vi "3D Hydrogen.vi"(9 "Z-Position":dbl format="%#_13g") -> (1 "reference out":refnum<vi>)   [LabVIEW 2023]
uses:
  <vilib>/picture/3D Picture Control/Object/Create Object (name).vi
  <vilib>/picture/3D Picture Control/Object/Add Object (no reference).vi
  <vilib>/picture/3D Picture Control/NI_3D Picture Control.lvlib
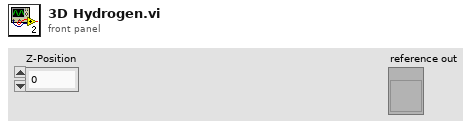
[diagram p1: front panel]
types:
  T1 = cluster{"Red":sgl, "Green":sgl, "Blue":sgl, "Alpha":sgl}
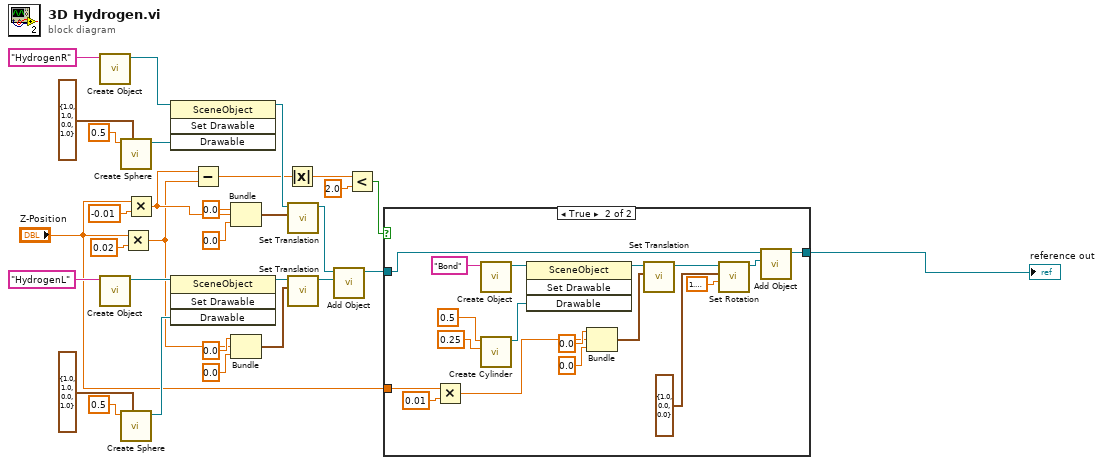
[diagram p0: block diagram]
diagram:
  n1 = call-poly <vilib>:"Create Object.vi"("Name"="HydrogenR") -> ("Scene:New Object"=w29:refnum<vi>)  [unwired: 9 in, 1 out]
  n2 = call-poly <vilib>:"Create Object.vi"("Name"="HydrogenL") -> ("Scene:New Object"=w24:refnum<vi>)  [unwired: 9 in, 1 out]
  n3 = call <vilib>:"Create Sphere.vi"("Color"=T1 {"Red"=1.0, "Green"=1.0, "Blue"=0.0, "Alpha"=1.0}, "Radius"=sgl 0.5) -> ("New Sphere Refnum"=w27:refnum<vi>)  [unwired: 8 in, 1 out]
  n4 = call <vilib>:"Create Sphere.vi"("Color"=T1 {"Red"=1.0, "Green"=1.0, "Blue"=0.0, "Alpha"=1.0}, "Radius"=sgl 0.5) -> ("New Sphere Refnum"=w22:refnum<vi>)  [unwired: 8 in, 1 out]
  n5 = Multiply(x="Z-Position", y=0.02) -> (x*y=w1:dbl)
  n6 = Multiply(x="Z-Position", y=-0.01) -> (x*y=w3:dbl)
  n7 = invoke class="SceneObject" method="Set Drawable"(reference=w29, "Drawable"=w27) -> (reference out=w13:refnum<vi>)  [unwired: 2 in, 3 out]
  n8 = invoke class="SceneObject" method="Set Drawable"(reference=w24, "Drawable"=w22) -> (reference out=w21:refnum<vi>)  [unwired: 2 in, 3 out]
  n9 = Subtract(x=w3, y=w1) -> (x-y=w6:dbl)
  n10 = Bundle(0.0, w3, 0.0) -> (w16:cluster{dbl, dbl, dbl})  [unwired: 1 in]
  n11 = Bundle(0.0, w1, 0.0) -> (w19:cluster{dbl, dbl, dbl})  [unwired: 1 in]
  n12 = Absolute Value(x=w6) -> (abs(x)=w8:dbl)
  n13 = call <vilib>:"Set Translation.vi"("Translation"=w16, "Scene Object"=w13) -> ("Translated Object"=w12:refnum<vi>)  [unwired: 8 in, 1 out]
  n14 = call <vilib>:"Set Translation.vi"("Translation"=w19, "Scene Object"=w21) -> ("Translated Object"=w20:refnum<vi>)  [unwired: 8 in, 1 out]
  n15 = call-poly <vilib>:"Add Object.vi"("New Object In"=w20, "Scene Object In"=w12) -> ("Scene Object Out"=w11:refnum<vi>)  [unwired: 8 in, 1 out]
  n16 = Less?(x=w8, y=2.0) -> (x < y?=w9:bool)
  n17 = case shown="True" w9 {
    tunnel: [w32 w44] -> w5
    tunnel: w11 -> [w32 w41]
    tunnel: "Z-Position" -> [_ w36]
    frame False {
    }
    frame True {
      n18 = Multiply(x=w36, y=0.01) -> (x*y=w33:dbl)
      n19 = call-poly <vilib>:"Create Object.vi"("Name"="Bond") -> ("Scene:New Object"=w49:refnum<vi>)  [unwired: 9 in, 1 out]
      n20 = call <vilib>:"Create Cylinder.vi"("Radius"=sgl 0.25, "Height"=sgl 0.5) -> ("New Cylinder Refnum"=w50:refnum<vi>)  [unwired: 8 in, 1 out]
      n21 = invoke class="SceneObject" method="Set Drawable"(reference=w49, "Drawable"=w50) -> (reference out=w45:refnum<vi>)  [unwired: 2 in, 3 out]
      n22 = Bundle(0.0, w33, 0.0) -> (w37:cluster{dbl, dbl, dbl})  [unwired: 1 in]
      n23 = call <vilib>:"Set Translation.vi"("Translation"=w37, "Scene Object"=w45) -> ("Translated Object"=w40:refnum<vi>)  [unwired: 8 in, 1 out]
      n24 = call <vilib>:"Set Rotation.vi"("Angle"=1.5707963267948966, "Axis"=cluster{"X":sgl, "Y":sgl, "Z":sgl} {"X"=1.0, "Y"=0.0, "Z"=0.0}, "Scene Object"=w40) -> ("Rotated Scene Object"=w42:refnum<vi>)  [unwired: 7 in, 1 out]
      n25 = call-poly <vilib>:"Add Object.vi"("New Object In"=w42, "Scene Object In"=w41) -> ("Scene Object Out"=w44:refnum<vi>)  [unwired: 8 in, 1 out]
    }
  }
  "reference out" <- w5
